vi "Release Priority Queue.vi"(8 "error in (no error)":errorcluster, 9 "Force Destroy? (F)":bool, 11 "Priority Queue":T1) -> (0 "error out":errorcluster)   [LabVIEW 2017, in "Communicable State Machine.lvlib"]
doc: "### Release Priority Queue.vi\n\n-- <b>Controls</b> --\n- <b>force destroy? (F)</b>:\n- <b>Priority Queue</b>:"
uses:
  Communicable State Machine.lvlib
  Priority Queue.ctl
  Typedef/_Cross CSM State Data.ctl
  Typedef/_CSM_MSG_TYPE.ctl
  Typedef/_Cross CSM State Response.ctl
  Typedef/_CSM_Response Source Message.ctl
  def-Data(LowPRI-Q).ctl
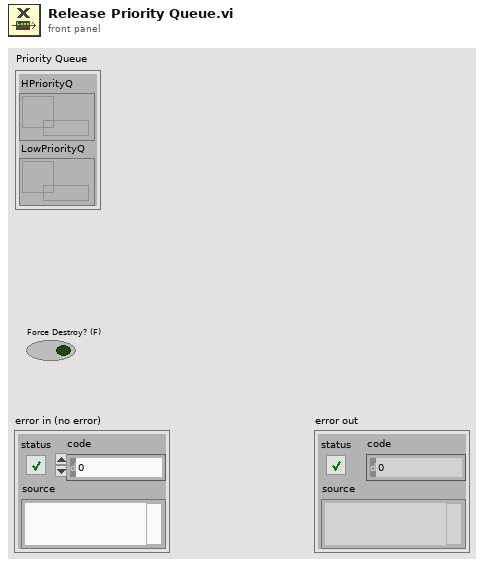
[diagram p1: front panel]
types:
  T1 = typedef "Communicable State Machine.lvlib/Priority Queue.ctl" = cluster{"HPriorityQ":refnum<queue>, "LowPriorityQ":refnum<queue>}
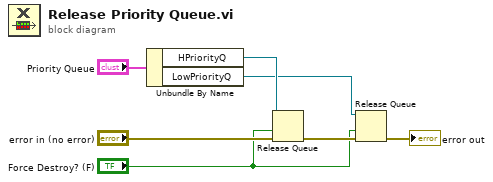
[diagram p0: block diagram]
diagram:
  n1 = Unbundle By Name("Priority Queue") -> ("HPriorityQ"=w6:refnum<queue>, "LowPriorityQ"=w5:refnum<queue>)
  n2 = Release Queue(queue=w6, force destroy? (F)="Force Destroy? (F)", error in (no error)="error in (no error)") -> (error out=w3:errorcluster)  [unwired: 2 out]
  n3 = Release Queue(queue=w5, force destroy? (F)="Force Destroy? (F)", error in (no error)=w3) -> (error out=→"error out":errorcluster)  [unwired: 2 out]
